vi "78020021.vi"() -> ()   [LabVIEW 2015]
doc: "Stand alone application to manage job dispatch of the modeler while displaying the status of jobs waiting, in-process or complete. Once a job is complete it is moved to the output buffer"
panel:
  out "Job Result":string
  out "TCP/IP Error":errorcluster
  out "Message":string
  out "Connect":errorcluster
  out "Consumed Count":i32
  out "state":string
  out "Computing Buffer":T1(array[cluster])
  out "Retry":u32
  out "Status Board":string[][](array[string])
  out "cmd line":string
  out "error out":errorcluster
  in  "Exit":bool
  in  "error in":errorcluster
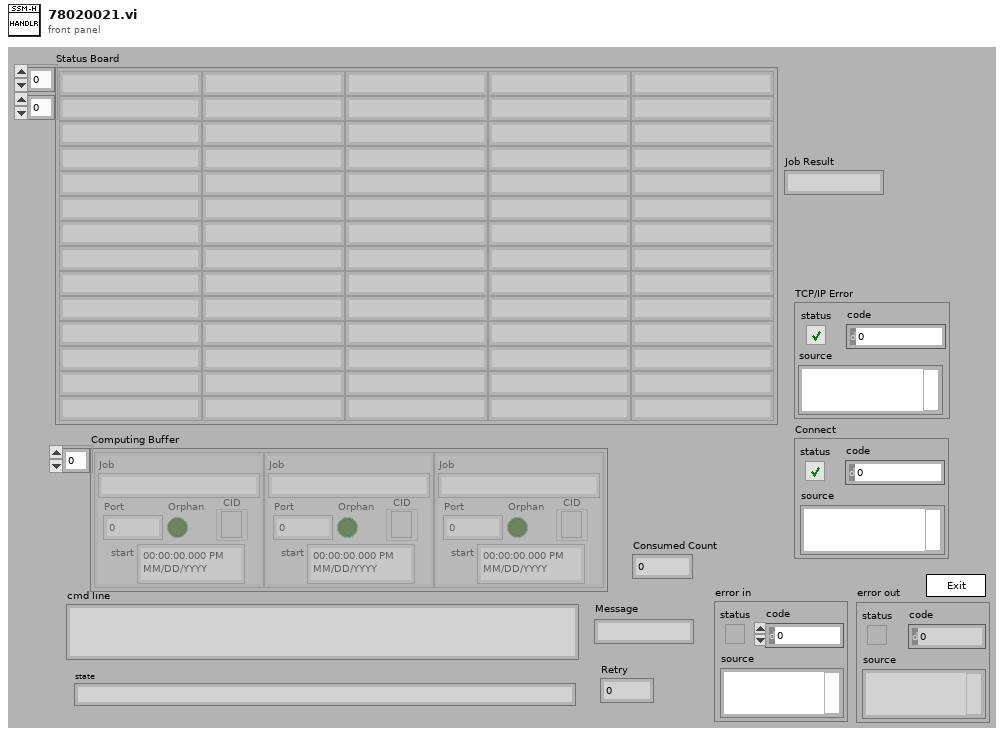
[diagram p1: front panel]
types:
  T1 = cluster{"Job":string, "Port":i32, "CID":refnum<k5>, "Orphan":bool, "start":timestamp}[]
  T2 = typedef "Rendezvous RefNum" = refnum<k1>
  T3 = cluster{"general":cluster{"project directory":path, "User Name":string, "User Level":string, "valid login":bool, "screen size":i32, "Screen Width":i32, "Screen Height":i32, "Login Password":string, "Login User Name":string, ".ini Resources":string[], "Control Refs":refnum<vi>[], "Error Ref out":refnum<vi>}, "rendezvous":T2, "queues":cluster{"Main":refnum<queue>, "Error":refnum<queue>, "VFP":refnum<queue>, "STATUS":refnum<queue>}, "NI Testand Config":cluster{"NI_Teststand DB":string[][]}, "Test Station Config":cluster{"Test Station DB":string[][], "Button Names":string[], "Short-cut keys":string[], "Paths to vis":path[], "Sub-Panel":bool[], "Wait until done":bool[], "Delay":i32[], "Dispose Ref":bool[], "Var. 1":string[], "Var. 2":string[], "Descriptions":string[], "Show Button":bool[], "Short-cut from DB":string[], "Prefix":string[]}, "Sub Panel":cluster{"Position":cluster{"Left":i32, "Top":i32}, "Hidden Pos":cluster{"Left":i32, "Top":i32}}, "Paths":cluster{"Upload":path, "Processing":path, "Repository":path, "Finished":path, "Error":path, "Modelers":path}, "Uploaded Jobs":cluster{"Name":string, "Files":i32}[], "Waiting Jobs":string[], "InProcess Jobs":string[], "Compute Engine":cluster{"EXE":string, "Start Port":i32, "Execution Limit":i32, "Log":string, "Max Time Sec":dbl}, "Computing Buffer":cluster{"Job":string, "Port":i32, "CID":refnum<k5>, "Orphan":bool, "start":timestamp}[], "Slot Open?":bool, "Retry":u32, "CPU Cores":string, "StatusBoard":path, "Retry Delay":dbl}
  T4 = enum32{"Invalid", "Standard", "Closed", "Hidden", "Minimized", "Maximized"}
  T5 = cluster{"status":bool, "code":i32, "resource not found":string}
  T6 = cluster{"Job":string, "Port":i32, "CID":refnum<k5>, "Orphan":bool, "start":timestamp}
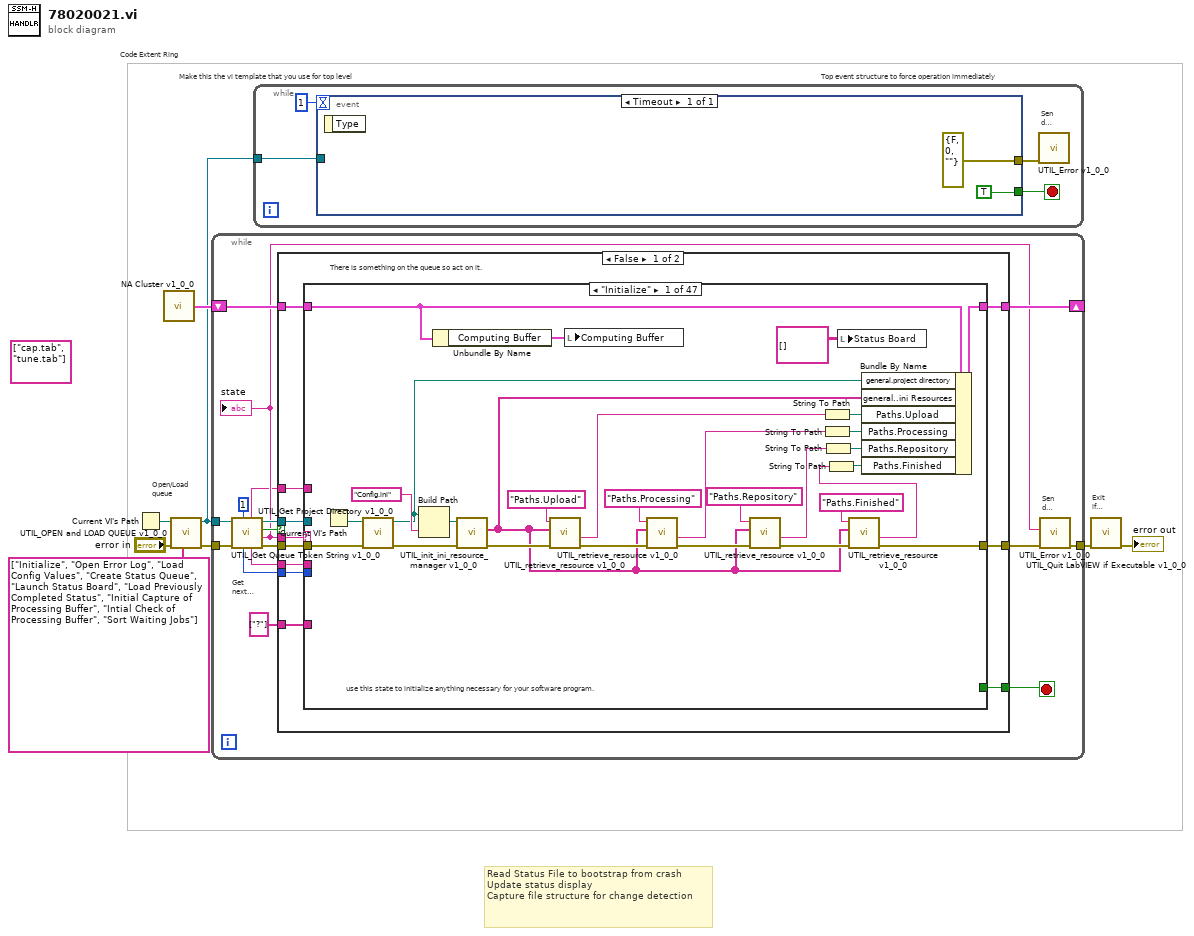
[diagram p0: block diagram]
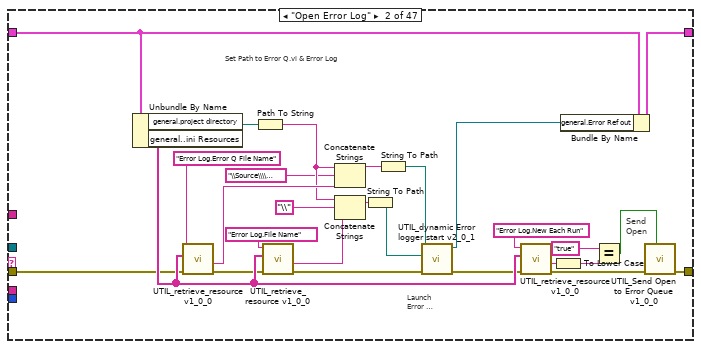
[diagram p2: hidden frame]
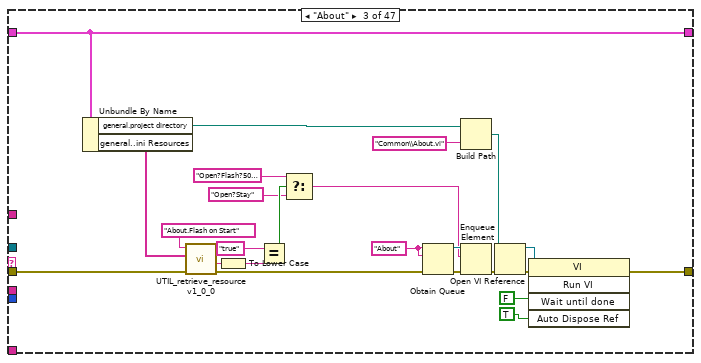
[diagram p3: hidden frame]
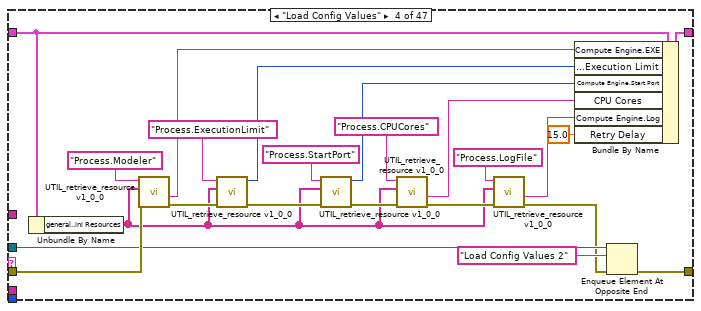
[diagram p4: hidden frame]
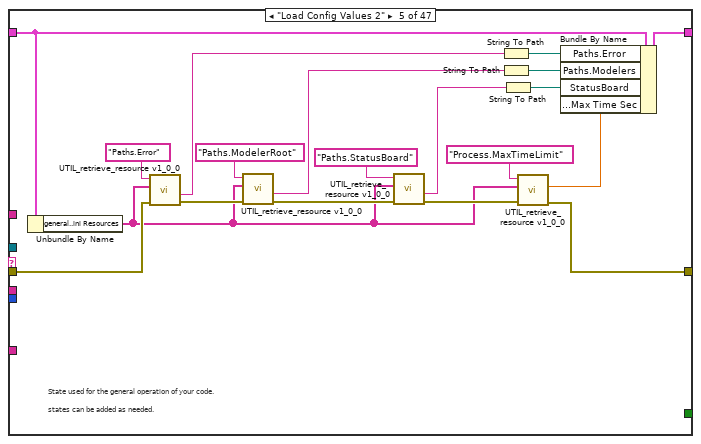
[diagram p5: hidden frame]
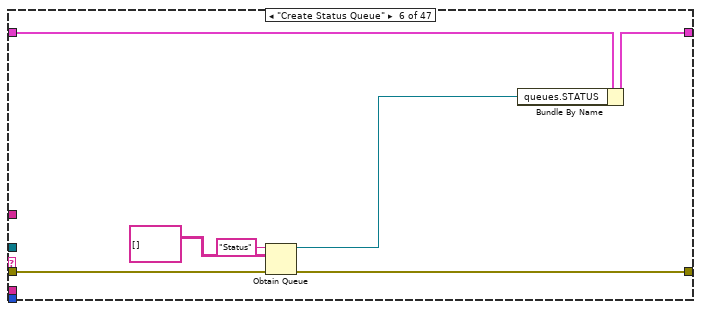
[diagram p6: hidden frame]
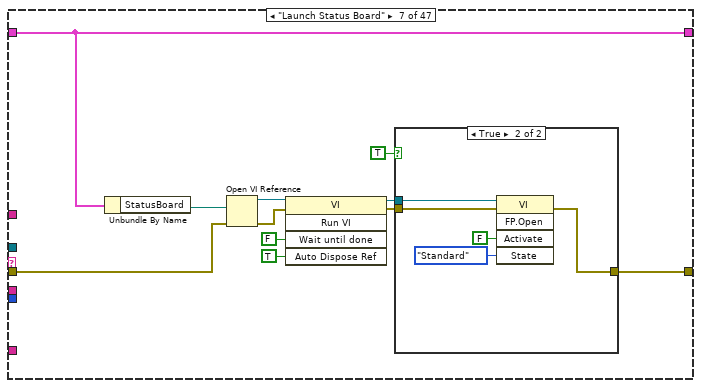
[diagram p7: hidden frame]
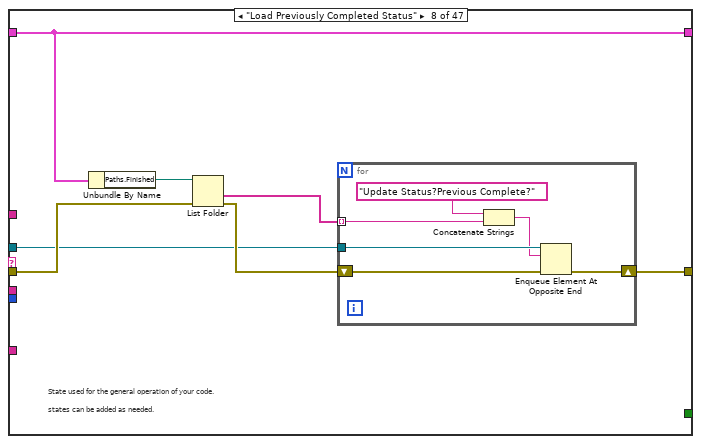
[diagram p9: hidden frame]
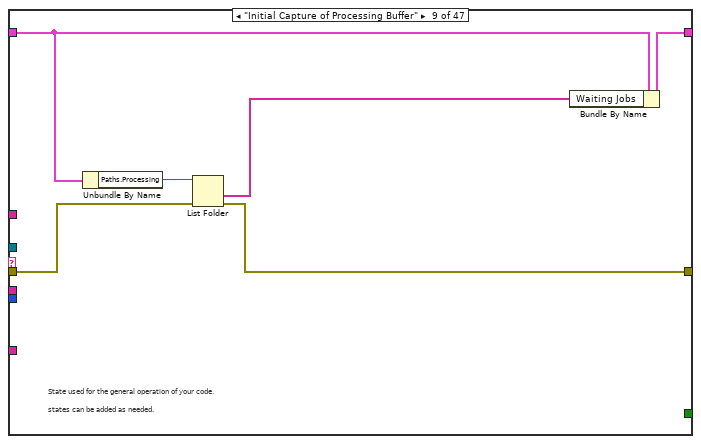
[diagram p10: hidden frame]
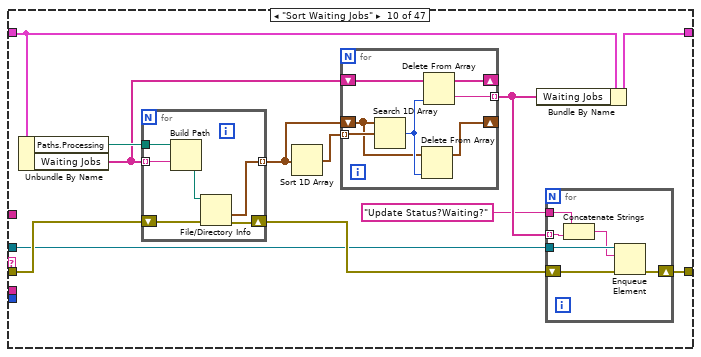
[diagram p11: hidden frame]
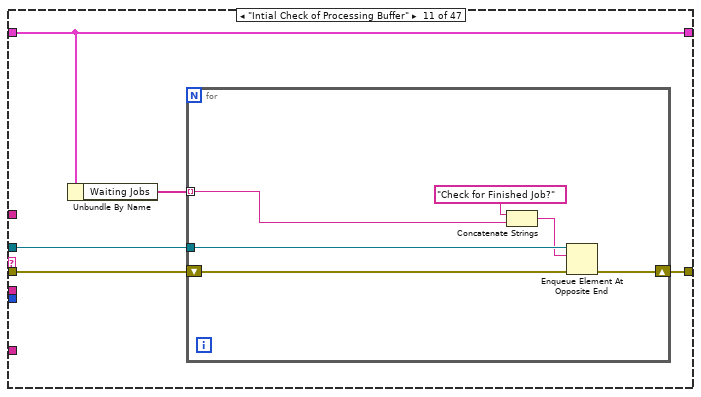
[diagram p12: hidden frame]
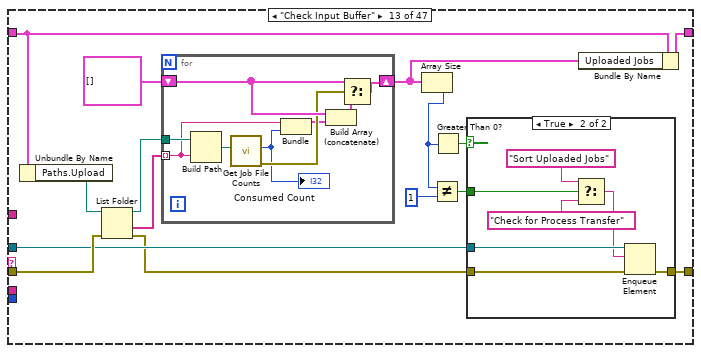
[diagram p14: hidden frame]
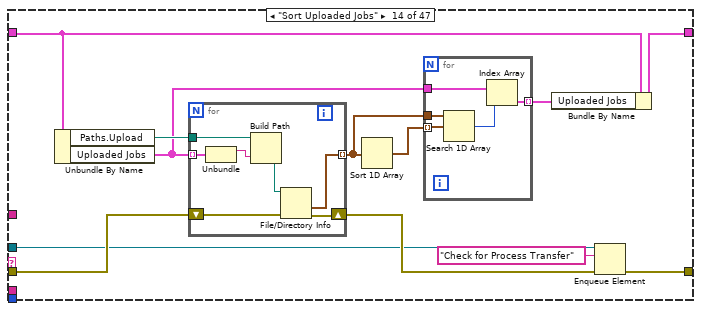
[diagram p16: hidden frame]
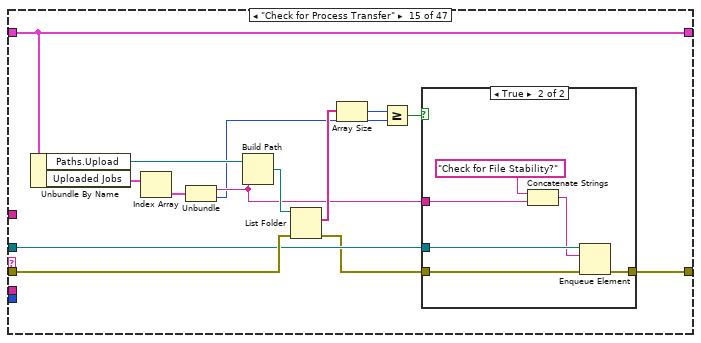
[diagram p17: hidden frame]
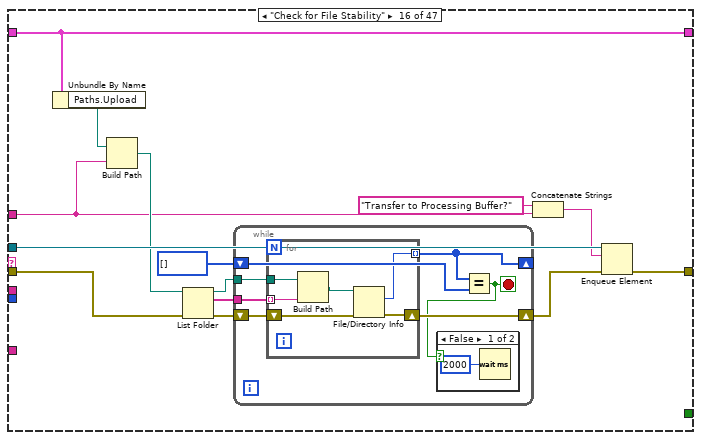
[diagram p19: hidden frame]
diagram:
  (unwired) string[] ["cap.tab", "tune.tab"]
  # "Read Status File to bootstrap from crash\nUpdate status display\nCapture file structure for change detection"
  # "Top event structure to force operation immediately"
  # "Open/Load\nqueue"
  # "Exit if\n.exe"
  # "Code Extent Ring"
  # "Make this the vi template that you use for top level"
  n1 = Current VI's Path() -> (path=w1:path)
  n2 = call "NA Cluster v1_0_0.vi"() -> ("FVP  MAIN"=w3:T3)
  n3 = call "UTIL_OPEN and LOAD QUEUE v1_0_0.vi"("Queue elements"=string[] ["Initialize", "Open Error Log", "Load Config Values", "Create Status Queue", "Launch Status Board", "Load Previously Completed Status", "Initial Capture of Processing Buffer", "Intial Check of Processing Buffer", "Sort Waiting Jobs"], "error in (no error)"="error in", "Path"=w1) -> ("error out"=w8:errorcluster, "Queue out"=w2:refnum<queue>)  [unwired: 1 in, 6 out]
  n4 = while {
    tunnel: w2 -> [w17]
    tunnel: w8 -> [w18]
    shift-right: [w23] -> _
    shift-left: w3 -> [w24]
    tunnel: [w20] -> w5
    stop <- w22 stop-if-true
    # "Get next\nstate"
    # "Send\nError"
    n5 = call "UTIL_Get Queue Token String v1_0_0.vi"("timeout in ms (-1)"=1, "error in (no error)"=w18, "queue"=w17) -> ("error out"=w19:errorcluster, "token string"=w11:string, "timed out?"=w12:bool, "queue out"=w13:refnum<queue>, "dup string"=w14:string, "dup - token string"=w10:string, "offset past token"=w15:i32)  [unwired: 1 in, 1 out]
    "state" <- w11
    n6 = case shown="False" w12 {
      tunnel: w13 -> [w34 w1091]
      tunnel: w19 -> [w35 w1093]
      tunnel: [w33 w1092] -> w21
      tunnel: w24 -> [w31 w1095]
      tunnel: [w32 w1094] -> w23
      tunnel: [w30 _] -> w22
      tunnel: w14 -> [w28 _]
      tunnel: w15 -> [w29 _]
      tunnel: w11 -> [w27 _]
      tunnel: w10 -> [w26 _]
      tunnel: string[] ["?"] -> [w25 _]
      frame False {
        # "There is something on the queue so act on it."
        n7 = case shown="\"Initialize\"" w27 {
          tunnel: w35 -> [w62 w64 w97 w133 w148 w163 w174 w187 w197 w209 w235 w242 w256 w285 w313 w334 w360 w372 w387 w408 w413 w431 w485 w592 w601 w617 w662 w698 w738 w758 w764 w774 w805 w819 w841 w877 w885 w907 w919 w944 w976 w1018 w1041 w1049 w1076 w1082 w1088]
          tunnel: w34 -> [_ _ _ w123 _ _ _ w183 _ w201 w232 _ w250 w279 w309 w327 w355 w362 w391 _ w414 w429 _ _ w602 w616 w653 w694 w737 w757 _ w773 w810 w836 w852 w883 _ w902 w909 w947 w979 w1008 w1036 w1050 w1077 w1081 _]
          tunnel: [w52 w90 w102 w124 w138 w162 w165 w184 w194 w204 w234 w242 w251 w280 w312 w329 w356 w367 w392 w408 w412 w430 w484 w592 w600 w618 w655 w697 w743 w756 w764 w778 w809 w835 w853 w882 w885 w903 w914 w948 w980 w1013 w1037 w1051 w1074 w1079 w1088] -> w33
          tunnel: w31 -> [w46 w73 w114 w135 w155 w159 w173 w182 w199 w211 w231 w243 w258 w287 w311 w323 w358 w375 w388 w409 w421 w432 w487 w593 w594 w613 w657 w685 w748 w760 w765 w767 w811 w837 w839 w884 w891 w905 w922 w940 w970 w1021 w1039 w1044 w1078 w1083 w1089]
          tunnel: [w63 w72 w114 w136 w154 w158 w173 w182 w198 w210 w231 w243 w257 w286 w311 w323 w358 w375 w390 w409 w420 w432 w487 w593 w594 w612 w657 w695 w751 w759 w765 w766 w811 w837 w839 w884 w890 w905 w922 w940 w970 w1021 w1039 w1043 w1078 w1083 w1089] -> w32
          tunnel: [_ _ _ _ _ _ _ _ _ _ _ _ _ _ _ _ _ _ _ _ _ _ _ _ _ _ _ _ _ _ _ _ _ _ _ _ _ _ _ _ _ _ _ _ _ TRUE _] -> w30
          tunnel: w29 -> [_ _ _ _ _ _ _ _ _ _ _ _ _ _ _ _ _ _ _ _ _ _ _ _ _ _ _ _ _ _ _ _ _ _ _ _ _ _ _ _ _ _ _ _ _ _ _]
          tunnel: w28 -> [_ _ _ _ _ _ _ _ _ _ _ _ _ _ _ _ _ _ _ _ _ _ w486 _ _ _ _ w690 _ _ _ _ _ _ _ _ _ _ _ _ _ _ _ _ _ _ w1086]
          tunnel: w26 -> [_ _ _ _ _ _ _ _ _ _ _ _ _ _ _ w321 w349 w361 w383 _ _ _ _ _ _ _ _ w691 w741 w754 _ w770 w807 w834 w840 w871 w887 w896 w908 w932 w962 w1007 w1030 w1042 _ _ _]
          tunnel: w25 -> [_ _ _ _ _ _ _ _ _ _ _ _ _ _ _ _ _ _ _ _ _ _ w472 _ _ _ _ _ _ _ _ _ _ _ _ _ _ _ _ _ _ _ _ _ _ _ _]
          frame "Initialize" {
            # "use this state to initialize anything necessary for your software program."
            n8 = Current VI's Path() -> (path=w61:path)
            n9 = call "UTIL_Get Project Directory v1_0_0.vi"("error in (no error)"=w62, "path"=w61) -> ("error out"=w59:errorcluster, "project directory"=w43:path)  [unwired: 8 out]
            n10 = Build Path(base path=w43, name or relative path="Config.ini") -> (appended path=w58:path)
            n11 = Unbundle By Name(w46) -> ("Computing Buffer"=w45:T1)
            n12 = call "UTIL_init_ini_resource_manager v1_0_0.vi"("error in"=w59, "Resource File"=w58) -> ("error out"=w56:errorcluster, "Resources"=w38:string[])  [unwired: 8 out]
            n13 = call "UTIL_retrieve_resource v1_0_0.vi"("error in"=w56, "Resources"=w38, "Resource Name"="Paths.Upload") -> ("error out"=w55:T5, "Resource String"=w50:string)  [unwired: 1 in, 6 out]
            n14 = local write "Computing Buffer"(w45) -> ()
            n15 = call "UTIL_retrieve_resource v1_0_0.vi"("error in"=w55, "Resources"=w38, "Resource Name"="Paths.Processing") -> ("error out"=w41:T5, "Resource String"=w51:string)  [unwired: 1 in, 6 out]
            n16 = call "UTIL_retrieve_resource v1_0_0.vi"("error in"=w41, "Resources"=w38, "Resource Name"="Paths.Repository") -> ("error out"=w40:T5, "Resource String"=w37:string)  [unwired: 1 in, 6 out]
            n17 = String To Path(string=w50) -> (path=w49:path)
            n18 = String To Path(string=w51) -> (path=w48:path)
            n19 = String To Path(string=w37) -> (path=w36:path)
            n20 = local write "Status Board"(string[][] [] ("Status Board")) -> ()
            n21 = call "UTIL_retrieve_resource v1_0_0.vi"("error in"=w40, "Resources"=w38, "Resource Name"="Paths.Finished") -> ("error out"=w52:T5, "Resource String"=w47:string)  [unwired: 1 in, 6 out]
            n22 = String To Path(string=w47) -> (path=w42:path)
            n23 = Bundle By Name(cluster=w46, "general.project directory"=w43, "general..ini Resources"=w38, "Paths.Upload"=w49, "Paths.Processing"=w48, "Paths.Repository"=w36, "Paths.Finished"=w42) -> (w63:T3)
          }
          frame "Open Error Log" {
            # "Launch\nError Q.vi"
            # "Send \nOpen"
            # "Set Path to Error Q.vi & Error Log"
            n24 = Unbundle By Name(w73) -> ("general.project directory"=w76:path, "general..ini Resources"=w87:string[])
            n25 = call "UTIL_retrieve_resource v1_0_0.vi"("error in"=w64, "Resources"=w87, "Resource Name"="Error Log.Error Q File Name") -> ("error out"=w86:T5, "Resource String"=w88:string)  [unwired: 1 in, 6 out]
            n26 = Path To String(path=w76) -> (string=w79:string)
            n27 = call "UTIL_retrieve_resource v1_0_0.vi"("error in"=w86, "Resources"=w87, "Resource Name"="Error Log.File Name") -> ("error out"=w68:T5, "Resource String"=w85:string)  [unwired: 1 in, 6 out]
            n28 = Concatenate Strings(w79, "\\Source\\\\UTIL\\" ("name or relative path"), w88) -> (w75:string)
            n29 = Concatenate Strings(w79, "\\" ("name or relative path"), w85) -> (w77:string)
            n30 = String To Path(string=w77) -> (path=w67:path)
            n31 = String To Path(string=w75) -> (path=w65:path)
            n32 = call "UTIL_dynamic Error logger start v2_0_1.vi"("error in (no error)"=w68, "Error File Path"=w67, "Error.vi Path"=w65) -> ("error out"=w69:errorcluster, "Error Ref out"=w66:refnum<vi>)  [unwired: 7 in]
            n33 = call "UTIL_retrieve_resource v1_0_0.vi"("error in"=w69, "Resources"=w87, "Resource Name"="Error Log.New Each Run") -> ("error out"=w71:T5, "Resource String"=w81:string)  [unwired: 1 in, 6 out]
            n34 = To Lower Case(string=w81) -> (all lower case string=w82:string)
            n35 = Bundle By Name(cluster=w73, "general.Error Ref out"=w66) -> (w72:T3)
            n36 = Equal?(x="true", y=w82) -> (x = y?=w70:bool)
            n37 = call "UTIL_Send Open to Error Queue v1_0_0.vi"("Append file? (False)"=w70, "error in (no error)"=w71) -> ("error out"=w90:errorcluster)  [unwired: 1 in, 8 out]
          }
          frame "About" {
            w106 = "About" ("name (unnamed)")
            n38 = Unbundle By Name(w114) -> ("general.project directory"=w105:path, "general..ini Resources"=w94:string[])
            n39 = call "UTIL_retrieve_resource v1_0_0.vi"("error in"=w97, "Resources"=w94, "Resource Name"="About.Flash on Start") -> ("error out"=w96:T5, "Resource String"=w99:string)  [unwired: 1 in, 6 out]
            n40 = To Lower Case(string=w99) -> (all lower case string=w100:string)
            n41 = Equal?(x="true", y=w100) -> (x = y?=w95:bool)
            n42 = Select(t="Open?Flash?5000" ("name (unnamed)"), s=w95, f="Open?Stay" ("name (unnamed)")) -> (s? t:f=w91:string)
            n43 = Obtain Queue(name (unnamed)=w106, element data type=w106, error in (no error)=w96) -> (queue out=w107:refnum<queue>, error out=w108:errorcluster)  [unwired: 2 in, 1 out]
            n44 = Build Path(base path=w105, name or relative path="Common\\About.vi" ("name (unnamed)")) -> (appended path=w103:path)
            n45 = Enqueue Element(queue=w107, element=w91, error in (no error)=w108) -> (error out=w111:errorcluster)  [unwired: 3 out]
            n46 = Open VI Reference(vi path=w103, error in (no error)=w111) -> (vi reference=w109:refnum<vi>, error out=w112:errorcluster)  [unwired: 4 out]
            n47 = invoke class="VI" method="Run VI"(reference=w109, error in=w112, "Wait until done"=FALSE ("Wait Until Done"), "Auto Dispose Ref"=TRUE ("Wait Until Done")) -> (error out=w102:errorcluster)  [unwired: 1 in, 4 out]
          }
          frame "Load Config Values" {
            n48 = Unbundle By Name(w135) -> ("general..ini Resources"=w118:string[])
            n49 = call "UTIL_retrieve_resource v1_0_0.vi"("error in"=w133, "Resources"=w118, "Resource Name"="Process.Modeler") -> ("error out"=w128:T5, "Resource String"=w132:string)  [unwired: 1 in, 6 out]
            n50 = call "UTIL_retrieve_resource v1_0_0.vi"("error in"=w128, "Resources"=w118, "Resource Name"="Process.ExecutionLimit") -> ("error out"=w127:T5, "Resource Integer"=w125:i32)  [unwired: 1 in, 6 out]
            n51 = call "UTIL_retrieve_resource v1_0_0.vi"("error in"=w127, "Resources"=w118, "Resource Name"="Process.StartPort") -> ("error out"=w130:T5, "Resource Integer"=w129:i32)  [unwired: 1 in, 6 out]
            n52 = call "UTIL_retrieve_resource v1_0_0.vi"("error in"=w130, "Resources"=w118, "Resource Name"="Process.CPUCores") -> ("error out"=w119:T5, "Resource String"=w121:string)  [unwired: 1 in, 6 out]
            n53 = call "UTIL_retrieve_resource v1_0_0.vi"("error in"=w119, "Resources"=w118, "Resource Name"="Process.LogFile") -> ("error out"=w120:T5, "Resource String"=w116:string)  [unwired: 1 in, 6 out]
            n54 = Bundle By Name(cluster=w135, "Compute Engine.EXE"=w132, "Compute Engine.Execution Limit"=w125, "Compute Engine.Start Port"=w129, "CPU Cores"=w121, "Compute Engine.Log"=w116, "Retry Delay"=15.0 ("Delay Time (s)")) -> (w136:T3)
            n55 = Enqueue Element At Opposite End(queue=w123, element="Load Config Values 2", error in (no error)=w120) -> (error out=w124:errorcluster)  [unwired: 1 in, 2 out]
          }
          frame "Load Config Values 2" {
            # "State used for the general operation of your code.\n\nstates can be added as needed."
            n56 = Unbundle By Name(w155) -> ("general..ini Resources"=w142:string[])
            n57 = call "UTIL_retrieve_resource v1_0_0.vi"("error in"=w148, "Resources"=w142, "Resource Name"="Paths.Error") -> ("error out"=w147:T5, "Resource String"=w146:string)  [unwired: 1 in, 6 out]
            n58 = call "UTIL_retrieve_resource v1_0_0.vi"("error in"=w147, "Resources"=w142, "Resource Name"="Paths.ModelerRoot") -> ("error out"=w150:T5, "Resource String"=w139:string)  [unwired: 1 in, 6 out]
            n59 = call "UTIL_retrieve_resource v1_0_0.vi"("error in"=w150, "Resources"=w142, "Resource Name"="Paths.StatusBoard") -> ("error out"=w143:T5, "Resource String"=w153:string)  [unwired: 1 in, 6 out]
            n60 = String To Path(string=w146) -> (path=w145:path)
            n61 = String To Path(string=w139) -> (path=w140:path)
            n62 = String To Path(string=w153) -> (path=w152:path)
            n63 = call "UTIL_retrieve_resource v1_0_0.vi"("error in"=w143, "Resources"=w142, "Resource Name"="Process.MaxTimeLimit") -> ("error out"=w138:T5, "Resource Number"=w141:dbl)  [unwired: 1 in, 6 out]
            n64 = Bundle By Name(cluster=w155, "Paths.Error"=w145, "Paths.Modelers"=w140, "StatusBoard"=w152, "Compute Engine.Max Time Sec"=w141) -> (w154:T3)
          }
          frame "Create Status Queue" {
            n65 = Obtain Queue(name (unnamed)="Status", element data type=string[][] [], error in (no error)=w163) -> (queue out=w157:refnum<queue>, error out=w162:errorcluster)  [unwired: 2 in, 1 out]
            n66 = Bundle By Name(cluster=w159, "queues.STATUS"=w157) -> (w158:T3)
          }
          frame "Launch Status Board" {
            n67 = Unbundle By Name(w173) -> ("StatusBoard"=w172:path)
            n68 = Open VI Reference(vi path=w172, error in (no error)=w174) -> (vi reference=w171:refnum<vi>, error out=w169:errorcluster)  [unwired: 4 in]
            n69 = invoke class="VI" method="Run VI"(reference=w171, error in=w169, "Wait until done"=FALSE ("Wait Until Done"), "Auto Dispose Ref"=TRUE ("Auto Dispose Reference")) -> (reference out=w167:refnum<vi>, error out=w166:errorcluster)  [unwired: 1 in, 3 out]
            n70 = case shown="True" TRUE {
              tunnel: w167 -> [_ w178]
              tunnel: w166 -> [w175 w177]
              tunnel: [w175 w176] -> w165
              frame False {
              }
              frame True {
                n71 = invoke class="VI" method="FP.Open"(reference=w178, error in=w177, "Activate"=FALSE ("Activate?"), "State"=T4."Standard") -> (error out=w176:errorcluster)  [unwired: 1 in, 4 out]
              }
            }
          }
          frame "Load Previously Completed Status" {
            # "State used for the general operation of your code.\n\nstates can be added as needed."
            n72 = Unbundle By Name(w182) -> ("Paths.Finished"=w186:path)
            n73 = List Folder(path=w186, error in=w187) -> (folder names=w181:string[], error out=w185:errorcluster)  [unwired: 2 in, 2 out]
            n74 = for {
              tunnel: w183 -> [w191]
              shift-right: [w192] -> w184
              shift-left: w185 -> [w193]
              tunnel: w181 -> [w188] mode=indexing
              n75 = Concatenate Strings("Update Status?Previous Complete?", w188) -> (w189:string)
              n76 = Enqueue Element At Opposite End(queue=w191, element=w189, error in (no error)=w193) -> (error out=w192:errorcluster)  [unwired: 1 in, 2 out]
            }
          }
          frame "Initial Capture of Processing Buffer" {
            # "State used for the general operation of your code.\n\nstates can be added as needed."
            n77 = Unbundle By Name(w199) -> ("Paths.Processing"=w196:path)
            n78 = List Folder(path=w196, error in=w197) -> (folder names=w195:string[], error out=w194:errorcluster)  [unwired: 2 in, 2 out]
            n79 = Bundle By Name(cluster=w199, "Waiting Jobs"=w195) -> (w198:T3)
          }
          frame "Sort Waiting Jobs" {
            n80 = Unbundle By Name(w211) -> ("Paths.Processing"=w208:path, "Waiting Jobs"=w205:string[])
            n81 = for {
              shift-right: [w227] -> w203
              shift-left: w209 -> [w230]
              tunnel: w208 -> [w229]
              tunnel: w205 -> [w225] mode=indexing
              tunnel: [w226] -> w206 mode=indexing
              n82 = Build Path(base path=w229, name or relative path=w225) -> (appended path=w228:path)
              n83 = File/Directory Info(path=w228, error in=w230) -> (last mod=w226:timestamp, error out=w227:errorcluster)  [unwired: 5 out]
            }
            n84 = Sort 1D Array(array=w206) -> (sorted array=w207:timestamp[])
            n85 = for {
              tunnel: w207 -> [w224] mode=indexing
              tunnel: [w222] -> w202 mode=indexing
              shift-right: [w219] -> _
              shift-left: w206 -> [w220]
              shift-right: [w218] -> _
              shift-left: w205 -> [w223]
              n86 = Search 1D Array(1D array=w220, element=w224) -> (index of element=w221:i32)  [unwired: 1 in]
              n87 = Delete From Array(array=w220, index=w221) -> (array with subset deleted=w219:timestamp[])  [unwired: 1 in, 1 out]
              n88 = Delete From Array(array=w223, index=w221) -> (deleted portion=w222:string, array with subset deleted=w218:string[])  [unwired: 1 in]
            }
            n89 = Bundle By Name(cluster=w211, "Waiting Jobs"=w202) -> (w210:T3)
            n90 = for {
              shift-right: [w217] -> w204
              shift-left: w203 -> [w216]
              tunnel: w202 -> [w214] mode=indexing
              tunnel: w201 -> [w215]
              tunnel: "Update Status?Waiting?" ("string") -> [w212]
              n91 = Concatenate Strings(w212, w214) -> (w213:string)
              n92 = Enqueue Element(queue=w215, element=w213, error in (no error)=w216) -> (error out=w217:errorcluster)  [unwired: 1 in, 2 out]
            }
          }
          frame "Intial Check of Processing Buffer" {
            n93 = Unbundle By Name(w231) -> ("Waiting Jobs"=w233:string[])
            n94 = for {
              shift-right: [w241] -> w234
              shift-left: w235 -> [w237]
              tunnel: w233 -> [w236] mode=indexing
              tunnel: w232 -> [w240]
              n95 = Concatenate Strings("Check for Finished Job?", w236) -> (w238:string)
              n96 = Enqueue Element At Opposite End(queue=w240, element=w238, error in (no error)=w237) -> (error out=w241:errorcluster)  [unwired: 1 in, 2 out]
            }
          }
          frame "---------------------------" {
          }
          frame "Check Input Buffer" {
            n97 = Unbundle By Name(w258) -> ("Paths.Upload"=w255:path)
            n98 = List Folder(path=w255, error in=w256) -> (path out=w253:path, folder names=w254:string[], error out=w249:errorcluster)  [unwired: 2 in, 1 out]
            n99 = for {
              tunnel: w254 -> [w274] mode=indexing
              shift-right: [w272] -> w248
              shift-left: cluster{string, "Consumer Count":i32}[] [] -> [w273]
              tunnel: w253 -> [w275]
              n100 = Build Path(base path=w275, name or relative path=w274) -> (appended path=w271:path)
              n101 = call "Get Job File Counts.vi"("Job Folder"=w271) -> ("error out"=w270:errorcluster, "Consumed Count"=w269:i32)  [unwired: 8 in, 1 out]
              "Consumed Count" <- w269
              n102 = Bundle(w274, "Consumed Count"=w269) -> (w268:cluster{string, "Consumed Count":i32})  [unwired: 1 in]
              n103 = Build Array (concatenate)(w273, w268) -> (w267:cluster{string, "Consumed Count":i32}[])
              n104 = Select(t=w273, s=w270, f=w267) -> (s? t:f=w272:cluster{string, "Consumed Count":i32}[])
            }
            n105 = Array Size(array=w248) -> (size(s)=w246:i32)
            n106 = Not Equal?(x=w246, y=1) -> (x != y?=w244:bool)
            n107 = Greater Than 0?(x=w246) -> (x > 0?=w247:bool)
            n108 = case shown="True" w247 {
              tunnel: [w259 w266] -> w251
              tunnel: w250 -> [_ w264]
              tunnel: w249 -> [w259 w265]
              tunnel: w244 -> [_ w263]
              frame False {
              }
              frame True {
                n109 = Select(t="Sort Uploaded Jobs" ("element"), s=w263, f="Check for Process Transfer" ("element")) -> (s? t:f=w260:string)
                n110 = Enqueue Element(queue=w264, element=w260, error in (no error)=w265) -> (error out=w266:errorcluster)  [unwired: 1 in, 2 out]
              }
            }
            n111 = Bundle By Name(cluster=w258, "Uploaded Jobs"=w248) -> (w257:T3)
          }
          frame "Sort Uploaded Jobs" {
            n112 = Unbundle By Name(w287) -> ("Paths.Upload"=w284:path, "Uploaded Jobs"=w277:cluster{"Name":string, "Files":i32}[])
            n113 = for {
              shift-right: [w295] -> w281
              shift-left: w285 -> [w299]
              tunnel: w284 -> [w298]
              tunnel: w277 -> [w297] mode=indexing
              tunnel: [w294] -> w282 mode=indexing
              n114 = Unbundle(w297) -> ("Name"=w293:string)  [unwired: 1 out]
              n115 = Build Path(base path=w298, name or relative path=w293) -> (appended path=w296:path)
              n116 = File/Directory Info(path=w296, error in=w299) -> (last mod=w294:timestamp, error out=w295:errorcluster)  [unwired: 5 out]
            }
            n117 = Sort 1D Array(array=w282) -> (sorted array=w283:timestamp[])
            n118 = for {
              tunnel: w283 -> [w292] mode=indexing
              tunnel: w282 -> [w291]
              tunnel: w277 -> [w289]
              tunnel: [w288] -> w278 mode=indexing
              n119 = Search 1D Array(1D array=w291, element=w292) -> (index of element=w290:i32)  [unwired: 1 in]
              n120 = Index Array(array=w289, index=w290) -> (element=w288:cluster{"Name":string, "Files":i32})
            }
            n121 = Bundle By Name(cluster=w287, "Uploaded Jobs"=w278) -> (w286:T3)
            n122 = Enqueue Element(queue=w279, element="Check for Process Transfer", error in (no error)=w281) -> (error out=w280:errorcluster)  [unwired: 1 in, 2 out]
          }
          frame "Check for Process Transfer" {
            n123 = Unbundle By Name(w311) -> ("Paths.Upload"=w310:path, "Uploaded Jobs"=w308:cluster{"Name":string, "Files":i32}[])
            n124 = Index Array(array=w308) -> (element=w300:cluster{"Name":string, "Files":i32})  [unwired: 1 in]
            n125 = Unbundle(w300) -> ("Name"=w302:string, "Files"=w301:i32)
            n126 = Build Path(base path=w310, name or relative path=w302) -> (appended path=w305:path)
            n127 = List Folder(path=w305, error in=w313) -> (filenames=w307:string[], error out=w303:errorcluster)  [unwired: 2 in, 2 out]
            n128 = Array Size(array=w307) -> (size(s)=w306:i32)
            n129 = Greater Or Equal?(x=w306, y=w301) -> (x >= y?=w304:bool)
            n130 = case shown="True" w304 {
              tunnel: w309 -> [_ w320]
              tunnel: w303 -> [w314 w319]
              tunnel: [w314 w318] -> w312
              tunnel: w302 -> [_ w316]
              frame False {
              }
              frame True {
                n131 = Concatenate Strings("Check for File Stability?" ("string"), w316) -> (w315:string)
                n132 = Enqueue Element(queue=w320, element=w315, error in (no error)=w319) -> (error out=w318:errorcluster)  [unwired: 1 in, 2 out]
              }
            }
          }
          frame "Check for File Stability" {
            n133 = Unbundle By Name(w323) -> ("Paths.Upload"=w322:path)
            n134 = Build Path(base path=w322, name or relative path=w321) -> (appended path=w324:path)
            n135 = List Folder(path=w324, error in=w334) -> (path out=w331:path, filenames=w332:string[], error out=w333:errorcluster)  [unwired: 2 in, 1 out]
            n136 = while {
              shift-right: [w338] -> w328
              shift-left: w333 -> [w341]
              tunnel: w332 -> [w340]
              tunnel: w331 -> [w339]
              shift-right: [w336] -> _
              shift-left: i64[] [] -> [w337]
              stop <- w335 stop-if-true
              n137 = for {
                shift-right: [w344] -> w338
                shift-left: w341 -> [w346]
                tunnel: w340 -> [w348] mode=indexing
                tunnel: w339 -> [w347]
                tunnel: [w343] -> w336 mode=indexing
                n138 = Build Path(base path=w347, name or relative path=w348) -> (appended path=w345:path)
                n139 = File/Directory Info(path=w345, error in=w346) -> (size=w343:i64, error out=w344:errorcluster)  [unwired: 5 out]
              }
              n140 = Equal?(x=w336, y=w337) -> (x = y?=w335:bool)
              n141 = case shown="False" w335 {
                frame False {
                  n142 = Wait (ms)(milliseconds to wait=u32 2000) -> ()  [unwired: 1 out]
                }
                frame True {
                }
              }
            }
            n143 = Concatenate Strings("Transfer to Processing Buffer?" ("string"), w321) -> (w325:string)
            n144 = Enqueue Element(queue=w327, element=w325, error in (no error)=w328) -> (error out=w329:errorcluster)  [unwired: 1 in, 2 out]
          }
          frame "Transfer to Processing Buffer" {
            n145 = Unbundle By Name(w358) -> ("Paths.Upload"=w350:path, "Paths.Processing"=w359:path)
            n146 = Build Path(base path=w350, name or relative path=w349) -> (appended path=w351:path)
            n147 = Build Path(base path=w359, name or relative path=w349) -> (appended path=w352:path)
            n148 = Copy(8:w360, 10:w352, 11:w351) -> (0:w357:errorcluster)  [unwired: 2 in, 2 out]
            n149 = Concatenate Strings("Check Processing Transfer?" ("element"), w349) -> (w353:string)
            n150 = Enqueue Element(queue=w355, element=w353, error in (no error)=w357) -> (error out=w356:errorcluster)  [unwired: 1 in, 2 out]
          }
          frame "Check Processing Transfer" {
            n151 = Unbundle By Name(w375) -> ("Paths.Processing"=w373:path, "Paths.Upload"=w374:path)
            n152 = Build Path(base path=w373, name or relative path=w361) -> (appended path=w369:path)
            n153 = Build Path(base path=w374, name or relative path=w361) -> (appended path=w371:path)
            n154 = List Folder(path=w371, error in=w372) -> (filenames=w365:string[], error out=w370:errorcluster)  [unwired: 2 in, 2 out]
            n155 = List Folder(path=w369, error in=w370) -> (filenames=w366:string[], error out=w368:errorcluster)  [unwired: 2 in, 2 out]
            n156 = Equal?(x=w365, y=w366) -> (x = y?=w364:bool[])
            n157 = And Array Elements(Boolean array=w364) -> (logical AND=w363:bool)
            n158 = case shown="True" w363 {
              tunnel: w368 -> [w376 w382]
              tunnel: [w376 w381] -> w367
              tunnel: w362 -> [_ w380]
              tunnel: w361 -> [_ w379]
              frame False {
              }
              frame True {
                n159 = Concatenate Strings("Delete Job Folder From Input Buffer?", w379) -> (w377:string)
                n160 = Enqueue Element(queue=w380, element=w377, error in (no error)=w382) -> (error out=w381:errorcluster)  [unwired: 1 in, 2 out]
              }
            }
          }
          frame "Delete Job Folder From Input Buffer" {
            n161 = Unbundle By Name(w388) -> ("Waiting Jobs"=w389:string[], "Paths.Upload"=w386:path)
            n162 = Build Path(base path=w386, name or relative path=w383) -> (appended path=w384:path)
            n163 = case shown="True" TRUE {
              tunnel: [w394 w395] -> w392
              tunnel: w387 -> [w394 w406]
              tunnel: w384 -> [_ w405]
              tunnel: w383 -> [_ w396]
              tunnel: w391 -> [_ w400]
              tunnel: [w393 w404] -> w390
              tunnel: w389 -> [_ w403]
              tunnel: w388 -> [w393 w401]
              frame False {
              }
              frame True {
                w407 = TRUE  # entire hierarchy
                n164 = Delete(path (use dialog)=w405, entire hierarchy (F)=w407, error in=w406) -> (error out=w398:errorcluster)  [unwired: 2 in, 2 out]
                n165 = Concatenate Strings("Update Status?Waiting?" ("string"), w396) -> (w397:string)
                n166 = Build Array (concatenate)(w403, w396) -> (w402:string[])
                n167 = Bundle By Name(cluster=w401, "Waiting Jobs"=w402) -> (w404:T3)
                n168 = Enqueue Element(queue=w400, element=w397, error in (no error)=w398) -> (error out=w395:errorcluster)  [unwired: 1 in, 2 out]
              }
            }
          }
          frame "=================" {
          }
          frame "Monitor Compute Buffer" {
            n169 = Unbundle By Name(w421) -> ("Computing Buffer"=w418:T1, "Compute Engine.Execution Limit"=w422:i32)
            n170 = Enqueue Element(queue=w414, element="Check for Job Dispatch", error in (no error)=w413) -> (queue out=w415:refnum<queue>, error out=w416:errorcluster)  [unwired: 1 in, 1 out]
            n171 = Array Size(array=w418) -> (size(s)=w410:i32)
            n172 = Less?(x=w410, y=w422) -> (x < y?=w419:bool)
            n173 = Greater Than 0?(x=w410) -> (x > 0?=w411:bool)
            n174 = case shown="True" w411 {
              tunnel: w416 -> [w423 w427]
              tunnel: w415 -> [_ w426]
              tunnel: [w423 w425] -> w412
              frame False {
              }
              frame True {
                n175 = Enqueue Element At Opposite End(queue=w426, element="Query Job Status", error in (no error)=w427) -> (error out=w425:errorcluster)  [unwired: 1 in, 2 out]
              }
            }
            n176 = Bundle By Name(cluster=w421, "Slot Open?"=w419) -> (w420:T3)
          }
          frame "Query Job Status" {
            n177 = Unbundle By Name(w432) -> ("Computing Buffer"=w428:T1)
            n178 = for {
              tunnel: w429 -> [w438]
              shift-right: [w439] -> w430
              shift-left: w431 -> [w440]
              tunnel: w428 -> [w437] mode=indexing
              i -> [w433]
              n179 = Unbundle By Name(w437) -> ("Job"=w436:string, "CID"=w434:refnum<k5>)
              n180 = Not A Number/Path/Refnum?(number/path/refnum=w434) -> (NaN/Path/Refnum?=w435:bool)
              n181 = case shown="False" w435 {
                tunnel: w440 -> [w461 w465]
                tunnel: w434 -> [w460 _]
                tunnel: [w456 w464] -> w439
                tunnel: w438 -> [w455 w463]
                tunnel: w436 -> [w446 _]
                tunnel: w433 -> [w443 w466]
                frame False {
                  # "Compute engine is not communicating"
                  n182 = Number To Decimal String(number=w443) -> (decimal integer string=w442:string)  [unwired: 1 in]
                  n183 = TCP Write(connection ID=w460, data in="status", error in (no error)=w461, 9:5000 ("timeout ms (25000)")) -> (connection ID out=w458:refnum<k5>, error out=w451:errorcluster)  [unwired: 1 out]
                  "TCP/IP Error" <- w451
                  n184 = Not(x=w451) -> (.not. x?=w447:bool)
                  n185 = TCP Read(connection ID=w458, bytes to read=100, error in (no error)=w451, 9:5000 ("timeout ms (25000)")) -> (data out=w444:string)  [unwired: 1 in, 2 out]
                  "Message" <- w444
                  n186 = Concatenate Strings("Check Job Timeout?" ("string"), w442) -> (w441:string)
                  n187 = Concatenate Strings("Update Status?UpdateProgress?", w446, "?", w444) -> (w450:string)
                  n188 = Select(t=w450, s=w447, f=w441) -> (s? t:f=w449:string)
                  n189 = Enqueue Element At Opposite End(queue=w455, element=w449) -> (error out=w456:errorcluster)  [unwired: 2 in, 2 out]
                }
                frame True {
                  n190 = Number To Decimal String(number=w466) -> (decimal integer string=w467:string)  [unwired: 1 in]
                  n191 = Concatenate Strings("Check Job Timeout?" ("string"), w467) -> (w462:string)
                  n192 = Enqueue Element(queue=w463, element=w462, error in (no error)=w465) -> (error out=w464:errorcluster)  [unwired: 1 in, 2 out]
                }
              }
            }
          }
          frame "Update Status" {
            # "Job  Status  TimeStarted  TimeCompleted"
            n193 = Unbundle By Name(w487) -> ("queues.STATUS"=w483:refnum<queue>)
            n194 = Scan String For Tokens(6:w472, 9:w486) -> (2:w481:i32, 3:w482:string)  [unwired: 4 in, 2 out]
            n195 = Scan String For Tokens(6:w472, 8:w481, 9:w482) -> (1:w469:string, 2:w475:i32, 3:w476:string)  [unwired: 3 in, 1 out]
            n196 = Scan String For Tokens(6:w472, 8:w475, 9:w476) -> (1:w471:string, 2:w473:i32, 3:w474:string)  [unwired: 3 in, 1 out]
            n197 = Dequeue Element(queue=w483, timeout in ms (-1)=0, error in (no error)=w485) -> (queue out=w479:refnum<queue>, element=w478:string[][], error out=w480:errorcluster)  [unwired: 1 out]
            n198 = case shown="\"Dispatched\"" w469 {
              tunnel: w471 -> [_ w499 w507 w521 w534 w537 w573 w583 w590]
              tunnel: w478 -> [w488 w495 w502 w517 w527 w545 w568 w578 w588]
              tunnel: [w488 w498 w506 w520 w533 w546 w572 w582 w589] -> w477
              tunnel: w472 -> [_ _ _ _ w524 _ _ _ _]
              tunnel: w474 -> [_ _ _ _ w531 _ _ _ _]
              tunnel: w473 -> [_ _ _ _ w530 _ _ _ _]
              frame "", Default {
              }
              frame "Waiting" {
                w494 = ""
                # "Update Status?Waiting?JobName"
                n199 = Get Date/Time String(date format (0)=enum16{"short", "long", "abbreviated"}."short") -> (date string=w492:string, time string=w491:string)  [unwired: 2 in]
                n200 = Concatenate Strings(w492, " " ("string"), w491) -> (w489:string)
                n201 = Build Array(w499, "Waiting" ("element"), w489, w494, w494) -> (w496:string[])
                n202 = Build Array (concatenate)(w496, w495) -> (w498:string[][])
              }
              frame "Dispatched" {
                # "Update Status?Dispatched?Job"
                n203 = Index Array(array=w502, index (col)=0 ("disabled index (col)")) -> (element=w508:string[])  [unwired: 1 in]
                n204 = Search 1D Array(1D array=w508, element=w507) -> (index of element=w501:i32)  [unwired: 1 in]
                n205 = Index Array(array=w502, index (row)=w501) -> (element=w503:string[])  [unwired: 1 in]
                n206 = Replace Array Subset(array=w503, new element="Launching Modeler" ("new element/subarray"), index=1) -> (w504:string[])
                n207 = Replace Array Subset(array=w502, new element=w504, index (row)=w501) -> (w506:string[][])  [unwired: 1 in]
              }
              frame "Started" {
                # "Update Status?Started?Job"
                n208 = Index Array(array=w517, index (col)=0 ("disabled index (col)")) -> (element=w522:string[])  [unwired: 1 in]
                n209 = Search 1D Array(1D array=w522, element=w521) -> (index of element=w515:i32)  [unwired: 1 in]
                n210 = Get Date/Time String(date format (0)=enum16{"short", "long", "abbreviated"}."short") -> (date string=w513:string, time string=w512:string)  [unwired: 2 in]
                n211 = Index Array(array=w517, index (row)=w515) -> (element=w516:string[])  [unwired: 1 in]
                n212 = Concatenate Strings(w513, " " ("string"), w512) -> (w510:string)
                n213 = Replace Array Subset(array=w516, new element=w510, index=3) -> (w518:string[])
                n214 = Replace Array Subset(array=w517, new element=w518, index (row)=w515) -> (w520:string[][])  [unwired: 1 in]
              }
              frame "UpdateProgress" {
                # "Update Status?UpdateProgress?Job?Message"
                n215 = Scan String For Tokens(6:w524, 8:w530, 9:w531) -> (1:w525:string)  [unwired: 3 in, 3 out]
                n216 = Index Array(array=w527, index (col)=0 ("disabled index (col)")) -> (element=w535:string[])  [unwired: 1 in]
                n217 = Search 1D Array(1D array=w535, element=w534) -> (index of element=w526:i32)  [unwired: 1 in]
                n218 = Index Array(array=w527, index (row)=w526) -> (element=w528:string[])  [unwired: 1 in]
                n219 = Replace Array Subset(array=w528, new element=w525, index=1) -> (w529:string[])
                n220 = Replace Array Subset(array=w527, new element=w529, index (row)=w526) -> (w533:string[][])  [unwired: 1 in]
              }
              frame "Complete" {
                # "Update Status?Complete?Job"
                n221 = Index Array(array=w545, index (col)=0 ("disabled index (col)")) -> (element=w547:string[])  [unwired: 1 in]
                n222 = Get Date/Time String(date format (0)=enum16{"short", "long", "abbreviated"}."short") -> (date string=w543:string, time string=w542:string)  [unwired: 2 in]
                n223 = Search 1D Array(1D array=w547, element=w537) -> (index of element=w538:i32)  [unwired: 1 in]
                n224 = Concatenate Strings(w543, " " ("string"), w542) -> (w540:string)
                n225 = case shown="0.." w538 {
                  selector: w538 -> [_ w556]
                  tunnel: [w555 w565] -> w546
                  tunnel: w545 -> [w551 w562]
                  tunnel: w540 -> [w550 w561]
                  tunnel: "Complete" ("new element/subarray") -> [w553 w557]
                  tunnel: w537 -> [w554 _]
                  frame ..-1 {
                    w549 = "" ("element")
                    n226 = Build Array(w554, w553, w549, w549, w550) -> (w552:string[])
                    n227 = Build Array (concatenate)(w552, w551) -> (w555:string[][])
                  }
                  frame 0.. {
                    n228 = Index Array(array=w562, index (row)=w556) -> (element=w560:string[])  [unwired: 1 in]
                    n229 = Replace Array Subset(array=w560, new element=w557, index=1) -> (w559:string[])
                    n230 = Replace Array Subset(array=w559, new element=w561, index=4) -> (w563:string[])
                    n231 = Replace Array Subset(array=w562, new element=w563, index (row)=w556) -> (w565:string[][])  [unwired: 1 in]
                  }
                }
              }
              frame "TimedOut" {
                # "Update Status?TimedOut?Job"
                n232 = Index Array(array=w568, index (col)=0 ("disabled index (col)")) -> (element=w574:string[])  [unwired: 1 in]
                n233 = Search 1D Array(1D array=w574, element=w573) -> (index of element=w567:i32)  [unwired: 1 in]
                n234 = Index Array(array=w568, index (row)=w567) -> (element=w569:string[])  [unwired: 1 in]
                n235 = Replace Array Subset(array=w569, new element="Error - Time Limit" ("new element/subarray"), index=1) -> (w570:string[])
                n236 = Replace Array Subset(array=w568, new element=w570, index (row)=w567) -> (w572:string[][])  [unwired: 1 in]
              }
              frame "Error" {
                # "Update Status?TimedOut?Job"
                n237 = Index Array(array=w578, index (col)=0 ("disabled index (col)")) -> (element=w584:string[])  [unwired: 1 in]
                n238 = Search 1D Array(1D array=w584, element=w583) -> (index of element=w577:i32)  [unwired: 1 in]
                n239 = Index Array(array=w578, index (row)=w577) -> (element=w579:string[])  [unwired: 1 in]
                n240 = Replace Array Subset(array=w579, new element="Error " ("new element/subarray"), index=1) -> (w580:string[])
                n241 = Replace Array Subset(array=w578, new element=w580, index (row)=w577) -> (w582:string[][])  [unwired: 1 in]
              }
              frame "Previous Complete" {
                w586 = ""
                n242 = Build Array(w590, "Complete" ("element"), w586, w586, w586) -> (w587:string[])
                n243 = Build Array (concatenate)(w588, w587) -> (w589:string[][])
              }
            }
            n244 = Enqueue Element(queue=w479, element=w477, error in (no error)=w480) -> (error out=w484:errorcluster)  [unwired: 1 in, 2 out]
          }
          frame ">>>>>>>>>>>>>>>>>>>>>>" {
          }
          frame "Check for Job Dispatch" {
            n245 = Unbundle By Name(w594) -> ("Waiting Jobs"=w598:string[])
            n246 = Unbundle By Name(w594) -> ("Slot Open?"=w595:bool)
            n247 = Array Size(array=w598) -> (size(s)=w597:i32)
            n248 = Greater Than 0?(x=w597) -> (x > 0?=w596:bool)
            n249 = And(x=w595, y=w596) -> (x .and. y?=w599:bool)
            n250 = case shown="True" w599 {
              tunnel: w602 -> [w604 w609]
              tunnel: w601 -> [w605 w610]
              tunnel: [w603 w607] -> w600
              frame False {
                n251 = Enqueue Element(queue=w604, element="Check Input Buffer", error in (no error)=w605) -> (error out=w603:errorcluster)  [unwired: 1 in, 2 out]
              }
              frame True {
                n252 = Enqueue Element At Opposite End(queue=w609, element="Get Modeler Info" ("string"), error in (no error)=w610) -> (error out=w607:errorcluster)  [unwired: 1 in, 2 out]
              }
            }
          }
          frame "Get Modeler Info" {
            # "Defaut Modeler?"
            n253 = Unbundle By Name(w613) -> ("Compute Engine.EXE"=w611:string, "Paths.Modelers"=w619:path, "Paths.Processing"=w627:path, "Waiting Jobs"=w629:string[])
            n254 = Index Array(array=w629) -> (element=w628:string)  [unwired: 1 in]
            n255 = Build Path(base path=w627, name or relative path=w628) -> (appended path=w626:path)
            n256 = call "Find Job Configuration File.vi"("error in (no error)"=w617, "Job Folder"=w626) -> ("error out"=w624:errorcluster, "Config File"=w625:path)  [unwired: 7 in, 1 out]
            n257 = call "Read Key - XML.vi"("error in (no error)"=w624, "Key"="Modeler", "Section"="FileConfiguration", "XML file"=w625) -> ("error out"=w621:errorcluster, "Value String"=w620:string)  [unwired: 4 in, 2 out]
            n258 = case shown="No Error" w621 {
              tunnel: w620 -> [w633 _]
              tunnel: w619 -> [w634 _]
              tunnel: [w630 w637] -> w614
              tunnel: w611 -> [_ w637]
              frame No Error {
                n259 = Build Path(base path=w634, name or relative path=w633) -> (appended path=w632:path)
                n260 = Concatenate Strings(w633, ".exe" ("string")) -> (w635:string)
                n261 = Build Path(base path=w632, name or relative path=w635) -> (appended path=w631:path)
                n262 = Path To String(path=w631) -> (string=w630:string)
              }
              frame Error {
              }
            }
            n263 = Enqueue Element(queue=w616, element="Dispatch Job" ("string"), error in (no error)=w617) -> (error out=w618:errorcluster)  [unwired: 1 in, 2 out]
            n264 = Bundle By Name(cluster=w613, "Compute Engine.EXE"=w614) -> (w612:T3)
          }
          frame "Dispatch Job" {
            n265 = Unbundle By Name(w657) -> ("Computing Buffer"=w664:T1, "Compute Engine.Execution Limit"=w667:i32, "Compute Engine.Start Port"=w666:i32, "Compute Engine.EXE"=w643:string, "Paths.Processing"=w648:path, "Waiting Jobs"=w642:string[], "CPU Cores"=w641:string, "Compute Engine.EXE"=w640:string)
            n266 = Index Array(array=w642) -> (element=w645:string)  [unwired: 1 in]
            n267 = String To Path(string=w640) -> (path=w639:path)
            n268 = for {
              tunnel: w664 -> [w669] mode=indexing
              tunnel: [w668] -> w663 mode=indexing
              n269 = Unbundle By Name(w669) -> ("Port"=w668:i32)
            }
            n270 = for {
              N: w667 -> [_]
              tunnel: w666 -> [w675]
              tunnel: [w674] -> w665 mode=indexing
              i -> [w676]
              n271 = Add(x=w675, y=w676) -> (x+y=w674:i32)
            }
            n272 = Strip Path(path=w639) -> (stripped path=w638:path)  [unwired: 1 out]
            n273 = Build Path(base path=w648, name or relative path=w645) -> (appended path=w647:path)
            n274 = Path To String(path=w647) -> (string=w646:string)
            n275 = for {
              tunnel: w665 -> [w670] mode=indexing
              tunnel: w663 -> [w673]
              tunnel: [w670] -> w656
              stop <- w671 stop-if-true
              n276 = Search 1D Array(1D array=w673, element=w670) -> (index of element=w672:i32)  [unwired: 1 in]
              n277 = Less Than 0?(x=w672) -> (x < 0?=w671:bool)
            }
            n278 = Number To Decimal String(number=w656) -> (decimal integer string=w650:string)  [unwired: 1 in]
            n279 = Concatenate Strings(w643, " -d ", w646, " -s ", w650, " -p ", w641) -> (w659:string)
            "cmd line" <- w659
            n280 = Concatenate Strings("Check Job Start?" ("string"), w650, "?" ("string"), w645) -> (w651:string)
            n281 = call <vilib>:"System Exec.vi"("wait until completion? (T)"=FALSE, "error in (no error)"=w662, "working directory"=w638, "command line"=w659) -> ("error out"=w654:errorcluster)  [unwired: 4 in, 3 out]
            n282 = Enqueue Element(queue=w653, element=w651, error in (no error)=w654) -> (error out=w655:errorcluster)  [unwired: 1 in, 2 out]
          }
          frame "Check Job Start" {
            w678 = string[] ["?"]
            n283 = Unbundle By Name(w685) -> ("Computing Buffer"=w696:T1, "Retry Delay"=w682:dbl)
            n284 = Scan String For Tokens(6:w678, 9:w690) -> (2:w693:i32, 3:w692:string)  [unwired: 4 in, 2 out]
            n285 = call "Time Delay"("error in (no error)"=w698, "Delay Time (s)"=w682) -> ("error out"=w686:errorcluster)  [unwired: 9 in]
            n286 = Scan String For Tokens(6:w678, 8:w693, 9:w692) -> (2:w688:i32, 3:w689:string)  [unwired: 3 in, 2 out]
            n287 = Scan String For Tokens(6:w678, 8:w688, 9:w689) -> (1:w687:string)  [unwired: 3 in, 3 out]
            n288 = Decimal String To Number(string=w691, default (0L)=u16 0 ("default (0 I32)")) -> (number=w681:u16)  [unwired: 1 in, 1 out]
            n289 = TCP Open Connection(address="127.0.0.1", remote port or service name=w681, error in (no error)=w686) -> (connection ID=w683:refnum<k5>, error out=w684:errorcluster)  [unwired: 2 in]
            n290 = case shown="Error" w684 {
              selector: w684 -> [_ w720]
              tunnel: w683 -> [w714 _]
              tunnel: [w708 w728] -> w697
              tunnel: w696 -> [w703 _]
              tunnel: w681 -> [w713 _]
              tunnel: w685 -> [w711 w721]
              tunnel: [w710 w727] -> w695
              tunnel: w694 -> [w707 w718]
              tunnel: w687 -> [w705 w723]
              tunnel: w690 -> [_ w716]
              tunnel: "Update Status?Dispatched?" ("address") -> [_ w715]
              frame No Error {
                n291 = Get Date/Time In Seconds() -> (seconds since 1Jan1904=w699:timestamp)
                n292 = Index Array(array=w703) -> (element=w702:T6)  [unwired: 1 in]
                n293 = Bundle By Name(cluster=w702, "Port"=w713, "CID"=w714, "Job"=w705, "Orphan"=FALSE, "start"=w699) -> (w712:T6)
                n294 = Build Array (concatenate)(w703, w712) -> (w709:T1)
                "Computing Buffer" <- w709
                n295 = Bundle By Name(cluster=w711, "Retry"=u32 0, "Computing Buffer"=w709) -> (w710:T3)
                n296 = Concatenate Strings("Remove Job From Waiting List?" ("string"), w705) -> (w706:string)
                n297 = Enqueue Element At Opposite End(queue=w707, element=w706) -> (error out=w708:errorcluster)  [unwired: 2 in, 2 out]
              }
              frame Error {
                n298 = Unbundle By Name(w721) -> ("Retry"=w722:u32)
                "Retry" <- w722
                n299 = Concatenate Strings(w715, w716) -> (w717:string)
                n300 = Less Or Equal?(x=w722, y=u32 3) -> (x <= y?=w724:bool)
                n301 = Enqueue Element At Opposite End(queue=w718, element=w717) -> (queue out=w719:refnum<queue>)  [unwired: 2 in, 2 out]
                n302 = case shown="True" w724 {
                  tunnel: [w733 w736] -> w728
                  tunnel: w719 -> [w731 w735]
                  tunnel: w716 -> [_ w734]
                  tunnel: w723 -> [w730 _]
                  frame False {
                    n303 = Concatenate Strings("Register Orphan Job?" ("element"), w730) -> (w732:string)
                    n304 = Enqueue Element At Opposite End(queue=w731, element=w732) -> (error out=w733:errorcluster)  [unwired: 2 in, 2 out]
                  }
                  frame True {
                    n305 = Enqueue Element(queue=w735, element=w734) -> (error out=w736:errorcluster)  [unwired: 2 in, 2 out]
                  }
                }
                n306 = Increment(x=w722) -> (x+1=w726:u32)
                n307 = Bundle By Name(cluster=w721, "Retry"=w726) -> (w727:T3)
                "Connect" <- w720
              }
            }
          }
          frame "Register Orphan Job" {
            n308 = Unbundle By Name(w748) -> ("Computing Buffer"=w746:T1)
            n309 = Index Array(array=w746) -> (element=w752:T6)  [unwired: 1 in]
            n310 = Get Date/Time In Seconds() -> (seconds since 1Jan1904=w739:timestamp)
            n311 = Bundle By Name(cluster=w752, "Orphan"=TRUE, "start"=w739, "Job"=w741) -> (w747:T6)
            n312 = Build Array (concatenate)(w746, w747) -> (w742:T1)
            n313 = Bundle By Name(cluster=w748, "Retry Delay"=10.0, "Retry"=u32 0, "Computing Buffer"=w742) -> (w751:T3)
            n314 = local write "Computing Buffer"(w742) -> ()
            n315 = Concatenate Strings("Remove Job From Waiting List?" ("string"), w741) -> (w744:string)
            n316 = Enqueue Element(queue=w737, element=w744, error in (no error)=w738) -> (error out=w743:errorcluster)  [unwired: 1 in, 2 out]
          }
          frame "Remove Job From Waiting List" {
            # "Remove Job From Waiting List?Job"
            n317 = Unbundle By Name(w760) -> ("Waiting Jobs"=w762:string[])
            n318 = Search 1D Array(1D array=w762, element=w754) -> (index of element=w763:i32)  [unwired: 1 in]
            n319 = Delete From Array(array=w762, index=w763) -> (array with subset deleted=w761:string[])  [unwired: 1 in, 1 out]
            n320 = Bundle By Name(cluster=w760, "Waiting Jobs"=w761) -> (w759:T3)
            n321 = Concatenate Strings("Update Status?Started?" ("string"), w754) -> (w753:string)
            n322 = Enqueue Element(queue=w757, element=w753, error in (no error)=w758) -> (error out=w756:errorcluster)  [unwired: 1 in, 2 out]
          }
          frame "<<<<<<<<<<<<<<<<<<<<<<<<" {
          }
          frame "Check Job Timeout" {
            # "Compute engine NOT communicating"
            n323 = Unbundle By Name(w767) -> ("Computing Buffer"=w771:T1, "Compute Engine.Max Time Sec"=w780:dbl)
            n324 = Decimal String To Number(string=w770) -> (number=w768:i32)  [unwired: 2 in, 1 out]
            n325 = Index Array(array=w771, index=w768) -> (element=w772:T6)
            n326 = Unbundle By Name(w772) -> ("start"=w777:timestamp, "Job"=w769:string)
            n327 = Get Date/Time In Seconds() -> (seconds since 1Jan1904=w779:timestamp)
            n328 = Subtract(x=w779, y=w777) -> (x-y=w776:dbl)
            n329 = Greater?(x=w776, y=w780) -> (0:w775:bool)
            n330 = case shown="False" w775 {
              tunnel: w774 -> [w786 w798]
              tunnel: w773 -> [w784 w796]
              tunnel: [w785 w797] -> w778
              tunnel: w771 -> [_ w795]
              tunnel: w769 -> [w783 w793]
              tunnel: w768 -> [_ w794]
              tunnel: w767 -> [w787 w789]
              tunnel: [w787 w788] -> w766
              frame False {
                # "Check that the job completed normally"
                n331 = Concatenate Strings("Check for Finished Job?" ("string"), w783) -> (w781:string)
                n332 = Enqueue Element(queue=w784, element=w781, error in (no error)=w786) -> (error out=w785:errorcluster)  [unwired: 1 in, 2 out]
              }
              frame True {
                # "Time limit reached - Free the slot"
                n333 = Delete From Array(array=w795, index=w794) -> (array with subset deleted=w790:T1)  [unwired: 1 in, 1 out]
                n334 = Bundle By Name(cluster=w789, "Computing Buffer"=w790) -> (w788:T3)
                n335 = Concatenate Strings("Update Status?TimedOut?", w793) -> (w791:string)
                n336 = Enqueue Element(queue=w796, element=w791, error in (no error)=w798) -> (error out=w797:errorcluster)  [unwired: 1 in, 2 out]
              }
            }
          }
          frame "Check for Finished Job" {
            n337 = Unbundle By Name(w811) -> ("Compute Engine.Log"=w801:string, "Paths.Processing"=w808:path)
            n338 = Build Path(base path=w808, name or relative path=w807) -> (appended path=w806:path)
            n339 = List Folder(path=w806, error in=w805) -> (filenames=w802:string[], error out=w804:errorcluster)  [unwired: 2 in, 2 out]
            n340 = To Lower Case(string=w801) -> (all lower case string=w800:string)
            n341 = To Lower Case(string=w802) -> (all lower case string=w799:string[])
            n342 = Search 1D Array(1D array=w799, element=w800) -> (index of element=w803:i32)  [unwired: 1 in]
            n343 = case shown="0.." w803 {
              tunnel: w804 -> [w812 w818]
              tunnel: w810 -> [_ w817]
              tunnel: [w812 w816] -> w809
              tunnel: w807 -> [_ w814]
              frame ..-1 {
              }
              frame 0.. {
                n344 = Concatenate Strings("Check Data Log?" ("element"), w814) -> (w815:string)
                n345 = Enqueue Element At Opposite End(queue=w817, element=w815, error in (no error)=w818) -> (error out=w816:errorcluster)  [unwired: 1 in, 2 out]
              }
            }
          }
          frame "Check Data Log" {
            n346 = Unbundle By Name(w837) -> ("Compute Engine.Log"=w832:string, "Paths.Processing"=w833:path)
            n347 = Build Path(base path=w833, name or relative path=w834) -> (appended path=w831:path)
            n348 = Build Path(base path=w831, name or relative path=w832) -> (appended path=w830:path)
            n349 = call "Read Key - XML.vi"("error in (no error)"=w819, "Key"="result", "Section"="OverallResult", "XML file"=w830) -> ("Value String"=w829:string)  [unwired: 4 in, 3 out]
            "Job Result" <- w829
            n350 = To Lower Case(string=w829) -> (all lower case string=w828:string)
            n351 = Equal?(x="pass", y=w828) -> (x = y?=w824:bool)
            n352 = Select(t="Check Job File Count?" ("element"), s=w824, f="Record Job Error?" ("element")) -> (s? t:f=w822:string)
            n353 = Concatenate Strings(w822, w834) -> (w826:string)
            n354 = Enqueue Element At Opposite End(queue=w836, element=w826, error in (no error)=w819) -> (error out=w835:errorcluster)  [unwired: 1 in, 2 out]
          }
          frame "Check Job File Count" {
            # "Perform File Count Check"
            n355 = Unbundle By Name(w839) -> ("Paths.Processing"=w845:path)
            n356 = Build Path(base path=w845, name or relative path=w840) -> (appended path=w844:path)
            n357 = List Folder(path=w844, error in=w841) -> (path out=w843:path, filenames=w838:string[], error out=w842:errorcluster)  [unwired: 2 in, 1 out]
            n358 = call "Get Job File Counts.vi"("error in"=w842, "Job Folder"=w843) -> ("error out"=w849:errorcluster, "Produced Count"=w851:i32, "Consumed Count"=w850:i32)  [unwired: 7 in]
            n359 = Array Size(array=w838) -> (size(s)=w847:i32)
            n360 = Add(x=w850, y=w851) -> (x+y=w848:i32)
            n361 = Greater Or Equal?(x=w847, y=w848) -> (x >= y?=w846:bool)
            n362 = case shown="True" w846 {
              tunnel: w849 -> [w859 w863]
              tunnel: w852 -> [w858 w864]
              tunnel: [w857 w868] -> w853
              tunnel: w840 -> [w855 w860]
              frame False {
                n363 = Concatenate Strings("Record Job Error?" ("element"), w855) -> (w856:string)
                n364 = Enqueue Element At Opposite End(queue=w858, element=w856, error in (no error)=w859) -> (error out=w857:errorcluster)  [unwired: 1 in, 2 out]
              }
              frame True {
                n365 = Concatenate Strings("Remove Job From Computing Buffer?" ("element"), w860) -> (w869:string)
                n366 = Concatenate Strings("Transfer to Archive Buffer?" ("element"), w860) -> (w861:string)
                n367 = Enqueue Element At Opposite End(queue=w864, element=w861, error in (no error)=w863) -> (queue out=w865:refnum<queue>, error out=w866:errorcluster)  [unwired: 1 in, 1 out]
                n368 = Enqueue Element At Opposite End(queue=w865, element=w869, error in (no error)=w866) -> (error out=w868:errorcluster)  [unwired: 1 in, 2 out]
              }
            }
          }
          frame "Record Job Error" {
            n369 = Concatenate Strings("Update Status?Error?" ("string"), w871) -> (w879:string)
            n370 = Enqueue Element At Opposite End(queue=w883, element=w879, error in (no error)=w877) -> (queue out=w875:refnum<queue>, error out=w876:errorcluster)  [unwired: 1 in, 1 out]
            n371 = Concatenate Strings("Transfer To Error Buffer?" ("string"), w871) -> (w872:string)
            n372 = Enqueue Element At Opposite End(queue=w875, element=w872, error in (no error)=w876) -> (queue out=w874:refnum<queue>, error out=w873:errorcluster)  [unwired: 1 in, 1 out]
            n373 = Concatenate Strings("Remove Job From Computing Buffer?" ("element"), w871) -> (w881:string)
            n374 = Enqueue Element At Opposite End(queue=w874, element=w881, error in (no error)=w873) -> (error out=w882:errorcluster)  [unwired: 1 in, 2 out]
          }
          frame "Remove Job From Computing Buffer" {
            # "Remove Job From Computing Buffer?Job"
            n375 = Unbundle By Name(w891) -> ("Computing Buffer"=w889:T1)
            n376 = for {
              tunnel: w889 -> [w894] mode=indexing
              tunnel: [w893] -> w888 mode=indexing
              n377 = Unbundle By Name(w894) -> ("Job"=w893:string)
            }
            n378 = Search 1D Array(1D array=w888, element=w887) -> (index of element=w892:i32)  [unwired: 1 in]
            n379 = Delete From Array(array=w889, index=w892) -> (array with subset deleted=w886:T1)  [unwired: 1 in, 1 out]
            n380 = Bundle By Name(cluster=w891, "Computing Buffer"=w886) -> (w890:T3)
            n381 = local write "Computing Buffer"(w886) -> ()
          }
          frame "Transfer to Archive Buffer" {
            n382 = Unbundle By Name(w905) -> ("Paths.Processing"=w897:path, "Paths.Repository"=w906:path)
            n383 = Build Path(base path=w897, name or relative path=w896) -> (appended path=w898:path)
            n384 = Build Path(base path=w906, name or relative path=w896) -> (appended path=w899:path)
            n385 = Copy(8:w907, 9:TRUE ("overwrite (F)"), 10:w899, 11:w898) -> (0:w904:errorcluster)  [unwired: 1 in, 2 out]
            n386 = Concatenate Strings("Check Archive Transfer?" ("element"), w896) -> (w900:string)
            n387 = Enqueue Element At Opposite End(queue=w902, element=w900, error in (no error)=w904) -> (error out=w903:errorcluster)  [unwired: 1 in, 2 out]
          }
          frame "Check Archive Transfer" {
            n388 = Unbundle By Name(w922) -> ("Paths.Repository"=w920:path, "Paths.Processing"=w921:path)
            n389 = Build Path(base path=w920, name or relative path=w908) -> (appended path=w916:path)
            n390 = Build Path(base path=w921, name or relative path=w908) -> (appended path=w918:path)
            n391 = List Folder(path=w918, error in=w919) -> (filenames=w912:string[], error out=w917:errorcluster)  [unwired: 2 in, 2 out]
            n392 = List Folder(path=w916, error in=w917) -> (filenames=w913:string[], error out=w915:errorcluster)  [unwired: 2 in, 2 out]
            n393 = Equal?(x=w912, y=w913) -> (x = y?=w911:bool[])
            n394 = And Array Elements(Boolean array=w911) -> (logical AND=w910:bool)
            n395 = case shown="True" w910 {
              tunnel: w915 -> [w923 w929]
              tunnel: [w923 w928] -> w914
              tunnel: w909 -> [_ w927]
              tunnel: w908 -> [_ w926]
              frame False {
              }
              frame True {
                n396 = Concatenate Strings("Create Finished Job?", w926) -> (w924:string)
                n397 = Enqueue Element At Opposite End(queue=w927, element=w924, error in (no error)=w929) -> (error out=w928:errorcluster)  [unwired: 1 in, 2 out]
              }
            }
          }
          frame "Create Finished Job" {
            # "Dont error in case exists"
            n398 = Unbundle By Name(w940) -> ("Paths.Repository"=w949:path)
            n399 = Unbundle By Name(w940) -> ("Paths.Finished"=w939:path)
            n400 = Match Pattern(string=w932, regular expression="_") -> (before substring=w931:string)  [unwired: 1 in, 3 out]
            n401 = Build Path(base path=w949, name or relative path=w932) -> (appended path=w943:path)
            n402 = Build Path(base path=w939, name or relative path=w931) -> (appended path=w938:path)
            n403 = call "Get Configuration Transfer Filenames.vi"("error in (no error)"=w944, "Job Folder"=w943) -> ("error out"=w934:errorcluster, "Transfer Files"=w930:string[], "Job Files"=w942:string[], "Job Folder out"=w941:path)  [unwired: 6 in]
            n404 = Create Folder(path (use dialog)=w938, error in=w934) -> (created path=w937:path, error out=w935:errorcluster)  [unwired: 1 in, 1 out]
            n405 = for {
              tunnel: w942 -> [w952]
              tunnel: w941 -> [w960]
              shift-right: [w958] -> w936
              shift-left: w934 -> [w959]
              tunnel: w937 -> [w957]
              tunnel: w935 -> [_]
              tunnel: w930 -> [w953] mode=indexing
              n406 = Search 1D Array(1D array=w952, element=w953) -> (index of element=w951:i32)  [unwired: 1 in]
              n407 = Index Array(array=w952, index=w951) -> (element=w950:string)
              n408 = Build Path(base path=w957, name or relative path=w950) -> (appended path=w955:path)
              n409 = Build Path(base path=w960, name or relative path=w950) -> (appended path=w956:path)
              n410 = Copy(8:w959, 9:TRUE ("overwrite (F)"), 10:w955, 11:w956) -> (0:w958:errorcluster)  [unwired: 1 in, 2 out]
            }
            n411 = Concatenate Strings("Delete Job Folder From Process Buffer?", w932) -> (w945:string)
            n412 = Enqueue Element At Opposite End(queue=w947, element=w945, error in (no error)=w936) -> (error out=w948:errorcluster)  [unwired: 1 in, 2 out]
          }
          frame "Create Finished Job (Legacy)" {
            # "Dont error in case exists"
            n413 = Unbundle By Name(w970) -> ("Paths.Repository"=w981:path)
            n414 = Unbundle By Name(w970) -> ("Paths.Finished"=w969:path)
            n415 = Match Pattern(string=w962, regular expression="_") -> (before substring=w961:string)  [unwired: 1 in, 3 out]
            n416 = Build Path(base path=w981, name or relative path=w962) -> (appended path=w975:path)
            n417 = List Folder(path=w975, error in=w976) -> (path out=w971:path, filenames=w974:string[], error out=w964:errorcluster)  [unwired: 2 in, 1 out]
            n418 = Build Path(base path=w969, name or relative path=w961) -> (appended path=w968:path)
            n419 = To Lower Case(string=w974) -> (all lower case string=w973:string[])
            n420 = Create Folder(path (use dialog)=w968, error in=w964) -> (created path=w967:path, error out=w965:errorcluster)  [unwired: 1 in, 1 out]
            n421 = for {
              tunnel: w973 -> [w988] mode=indexing
              tunnel: ".tab" ("regular expression") -> [w991]
              tunnel: w971 -> [w989]
              shift-right: [w985] -> w966
              shift-left: w964 -> [w986]
              tunnel: w967 -> [w984]
              tunnel: w965 -> [_]
              n422 = Match Pattern(string=w988, regular expression=w991) -> (before substring=w983:string, offset past match=w990:i32)  [unwired: 1 in, 2 out]
              n423 = Greater Or Equal To 0?(x=w990) -> (x >= 0?=w987:bool)
              n424 = Reverse String(1:w983) -> (0:w982:string)
              n425 = case shown="True" w987 {
                tunnel: w989 -> [_ w1006]
                tunnel: w988 -> [_ w1001]
                tunnel: w986 -> [w992 w1005]
                tunnel: [w992 w1003] -> w985
                tunnel: w984 -> [_ w1002]
                tunnel: w982 -> [_ w998]
                frame False {
                }
                frame True {
                  n426 = Match Pattern(string=w998, regular expression="_") -> (before substring=w996:string)  [unwired: 1 in, 3 out]
                  n427 = Reverse String(1:w996) -> (0:w993:string)
                  n428 = Concatenate Strings(w993, ".tab" ("regular expression")) -> (w995:string)
                  n429 = Build Path(base path=w1002, name or relative path=w995) -> (appended path=w1000:path)
                  n430 = Build Path(base path=w1006, name or relative path=w1001) -> (appended path=w1004:path)
                  n431 = Copy(8:w1005, 9:TRUE ("overwrite (F)"), 10:w1000, 11:w1004) -> (0:w1003:errorcluster)  [unwired: 1 in, 2 out]
                }
              }
            }
            n432 = Concatenate Strings("Delete Job Folder From Process Buffer?", w962) -> (w977:string)
            n433 = Enqueue Element At Opposite End(queue=w979, element=w977, error in (no error)=w966) -> (error out=w980:errorcluster)  [unwired: 1 in, 2 out]
          }
          frame "Check Error Transfer" {
            n434 = Unbundle By Name(w1021) -> ("Paths.Error"=w1019:path, "Paths.Processing"=w1020:path)
            n435 = Build Path(base path=w1019, name or relative path=w1007) -> (appended path=w1015:path)
            n436 = Build Path(base path=w1020, name or relative path=w1007) -> (appended path=w1017:path)
            n437 = List Folder(path=w1017, error in=w1018) -> (filenames=w1011:string[], error out=w1016:errorcluster)  [unwired: 2 in, 2 out]
            n438 = List Folder(path=w1015, error in=w1016) -> (filenames=w1012:string[], error out=w1014:errorcluster)  [unwired: 2 in, 2 out]
            n439 = Equal?(x=w1011, y=w1012) -> (x = y?=w1010:bool[])
            n440 = And Array Elements(Boolean array=w1010) -> (logical AND=w1009:bool)
            n441 = case shown="True" w1009 {
              tunnel: w1014 -> [w1022 w1028]
              tunnel: [w1022 w1027] -> w1013
              tunnel: w1008 -> [_ w1026]
              tunnel: w1007 -> [_ w1025]
              frame False {
              }
              frame True {
                n442 = Concatenate Strings("Delete Job Folder From Process Buffer?", w1025) -> (w1023:string)
                n443 = Enqueue Element At Opposite End(queue=w1026, element=w1023, error in (no error)=w1028) -> (error out=w1027:errorcluster)  [unwired: 1 in, 2 out]
              }
            }
          }
          frame "Transfer To Error Buffer" {
            n444 = Unbundle By Name(w1039) -> ("Paths.Processing"=w1031:path, "Paths.Error"=w1040:path)
            n445 = Build Path(base path=w1031, name or relative path=w1030) -> (appended path=w1032:path)
            n446 = Build Path(base path=w1040, name or relative path=w1030) -> (appended path=w1033:path)
            n447 = Copy(8:w1041, 9:TRUE ("overwrite (F)"), 10:w1033, 11:w1032) -> (0:w1038:errorcluster)  [unwired: 1 in, 2 out]
            n448 = Concatenate Strings("Check Error Transfer?" ("element"), w1030) -> (w1034:string)
            n449 = Enqueue Element At Opposite End(queue=w1036, element=w1034, error in (no error)=w1038) -> (error out=w1037:errorcluster)  [unwired: 1 in, 2 out]
          }
          frame "Delete Job Folder From Process Buffer" {
            w1047 = TRUE  # Put some check here
            n450 = Unbundle By Name(w1044) -> ("Waiting Jobs"=w1045:string[], "Paths.Processing"=w1048:path)
            n451 = Build Path(base path=w1048, name or relative path=w1042) -> (appended path=w1046:path)
            n452 = case shown="True" w1047 {
              tunnel: [w1053 w1064] -> w1051
              tunnel: w1049 -> [w1053 w1054]
              tunnel: w1046 -> [_ w1065]
              tunnel: w1042 -> [_ w1055]
              tunnel: w1050 -> [_ w1063]
              tunnel: w1045 -> [_ w1057]
              tunnel: w1044 -> [w1052 w1060]
              tunnel: [w1052 w1059] -> w1043
              frame False {
              }
              frame True {
                w1066 = TRUE  # entire hierarchy
                # "only for startup"
                n453 = Search 1D Array(1D array=w1057, element=w1055) -> (index of element=w1058:i32)  [unwired: 1 in]
                n454 = Delete From Array(array=w1057, index=w1058) -> (array with subset deleted=w1056:string[])  [unwired: 1 in, 1 out]
                n455 = Delete(path (use dialog)=w1065, entire hierarchy (F)=w1066, error in=w1054) -> ()  [unwired: 2 in, 3 out]
                n456 = Concatenate Strings("Update Status?Complete?" ("string"), w1055) -> (w1062:string)
                n457 = Bundle By Name(cluster=w1060, "Waiting Jobs"=w1056) -> (w1059:T3)
                n458 = Enqueue Element At Opposite End(queue=w1063, element=w1062, error in (no error)=w1054) -> (error out=w1064:errorcluster)  [unwired: 1 in, 2 out]
              }
            }
          }
          frame "Clean Up" {
            w1073 = "Status Board" ("name (unnamed)")
            # "Exit\nError log"
            # "Cleanup state before Exiting"
            n459 = Enqueue Element(queue=w1077, element="Exit", error in (no error)=w1076) -> (error out=w1072:errorcluster)  [unwired: 3 out]
            n460 = Obtain Queue(name (unnamed)=w1073, element data type=w1073, create if not found? (T)=FALSE, error in (no error)=w1072) -> (queue out=w1069:refnum<queue>, error out=w1070:errorcluster)  [unwired: 1 in, 1 out]
            n461 = Enqueue Element(queue=w1069, element="Exit", error in (no error)=w1070) -> (error out=w1067:errorcluster)  [unwired: 1 in, 2 out]
            n462 = call "UTIL_Send Close to Error Queue v1_0_0.vi"("error in (no error)"=w1067) -> ("error out"=w1074:errorcluster)  [unwired: 1 in, 9 out]
          }
          frame "Exit" {
            # "Stop the state machine -->"
            # "Destroy\nQueue"
            # "Clean up outstanding references and Exit this software program."
            n463 = Release Queue(queue=w1081, force destroy? (F)=TRUE, error in (no error)=w1082) -> (error out=w1079:errorcluster)  [unwired: 2 out]
          }
          frame Default {
            # "State used to show developer that they have messed up state machine logic."
            n464 = Concatenate Strings("Error in Logic:\n\nYou should not see this.\n\nThis is what you sent:" ("message"), w1086) -> (w1085:string)
            n465 = One Button Dialog(message=w1085) -> ()  [unwired: 2 out]
          }
        }
      }
      frame True {
        # "Timeout set to -1 so event structure will not activate the timeout state of the event structure.\n Use -1 or \"other\" as needed."
        # "Queue Timed out.."
        n466 = event shown="[0] Timeout" {
          selector: _ -> [_ _]
          dyn-events: _ -> [_ _]
          timeout: 1000 -> [_ _]
          tunnel: [w1102 w1108] -> w1094
          tunnel: w1095 -> [w1102 w1108]
          tunnel: [w1096 w1104] -> w1092
          tunnel: w1093 -> [w1099 w1106]
          tunnel: w1091 -> [w1098 w1105]
          event Timeout {
            n467 = event-data() -> ()  [unwired: 3 out]
            n468 = Unbundle By Name(w1102) -> ("queues.STATUS"=w1101:refnum<queue>)
            n469 = Enqueue Element(queue=w1098, element="Monitor Compute Buffer", error in (no error)=w1099) -> (error out=w1096:errorcluster)  [unwired: 1 in, 2 out]
            n470 = Preview Queue Element(queue=w1101, timeout in ms (-1)=0) -> (element=→"Status Board":string[][])  [unwired: 1 in, 3 out]
          }
          event "Exit": Value Change {
            n471 = event-data() -> ()  [unwired: 7 out]
            n472 = Enqueue Element(queue=w1105, element="Clean Up", error in (no error)=w1106) -> (error out=w1104:errorcluster)  [unwired: 3 out]
          }
        }
      }
    }
    n473 = call "UTIL_Error v1_0_0.vi"("error in (no error)"=w21, "State"=w11) -> ("error out"=w20:errorcluster)  [unwired: 1 in, 8 out]
  }
  n474 = while {
    tunnel: w2 -> [w1112]
    stop <- w1111 stop-if-true
    # "Send\nError"
    n475 = event shown="[0] Timeout" {
      selector: _ -> [_]
      dyn-events: _ -> [_]
      timeout: 1 -> [_]
      tunnel: w1112 -> [_]
      tunnel: [TRUE ("Wait Until Done")] -> w1111
      tunnel: [errorcluster {"status"=FALSE, "code"=0, "source"=""} ("error in 2")] -> w1110
      event Timeout {
        n476 = event-data() -> ()  [unwired: 2 out]
      }
    }
    n477 = call "UTIL_Error v1_0_0.vi"("error in (no error)"=w1110) -> ()  [unwired: 2 in, 9 out]
  }
  n478 = call "UTIL_Quit LabVIEW if Executable v1_0_0.vi"("error in (no error)"=w5) -> ("error out"=→"error out":errorcluster)  [unwired: 9 out]
